vi "findbufferbyname.vi"(9 "buffer name":string, 10 "Buffers":T1[](array[typedef])) -> (1 "found":bool, 2 "buffer found":T1, 3 "index":i32)   [LabVIEW 2016]
uses:
  private/vis/BufferStruct.ctl
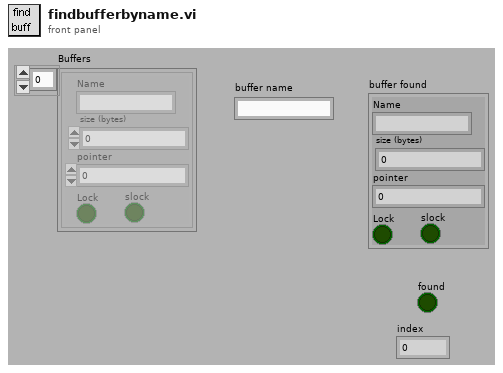
[diagram p1: front panel]
types:
  T1 = typedef "BufferStruct.ctl" = cluster{"Name":string, "size (bytes)":u64, "pointer":u64, "Lock":bool, "slock":bool}
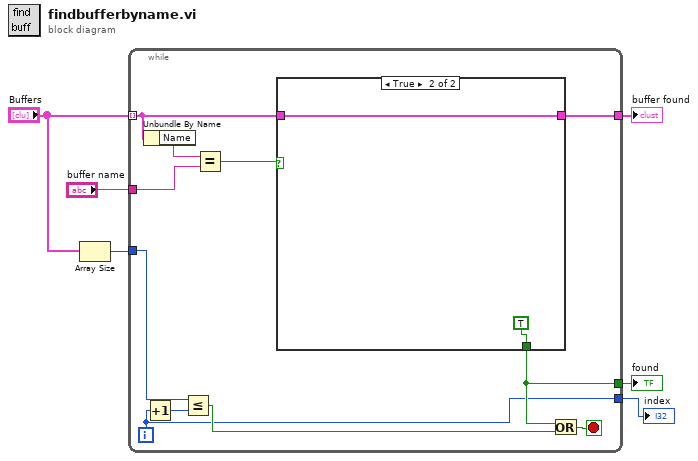
[diagram p0: block diagram]
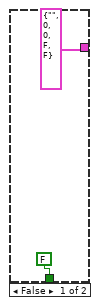
[diagram p2: hidden frame]
diagram:
  n1 = Array Size(array="Buffers") -> (size(s)=w4:i32)
  n2 = while {
    tunnel: [w7] -> w1
    tunnel: [w8] -> w2
    tunnel: [w9] -> w3
    tunnel: w4 -> [w13]
    tunnel: "buffer name" -> [w16]
    tunnel: "Buffers" -> [w14] mode=indexing
    i -> [w7]
    stop <- w11 stop-if-true
    n3 = Unbundle By Name(w14) -> ("Name"=w17:string)
    n4 = Increment(x=w7) -> (x+1=w12:i32)
    n5 = Less Or Equal?(x=w13, y=w12) -> (x <= y?=w10:bool)
    n6 = Equal?(x=w17, y=w16) -> (x = y?=w15:bool)
    n7 = case shown="True" w15 {
      tunnel: w14 -> [_ w20]
      tunnel: [FALSE TRUE] -> w9
      tunnel: [T1 {"Name"="", "size (bytes)"=0, "pointer"=0, "Lock"=FALSE, "slock"=FALSE} ("buffer") w20] -> w8
      frame False {
      }
      frame True {
      }
    }
    n8 = Or(x=w9, y=w10) -> (x .or. y?=w11:bool)
  }
  "found" <- w3
  "buffer found" <- w2
  "index" <- w1
